vi "Calculate Directions.vi"(8 "error in (no error)":errorcluster, 10 "Heading":T1, 11 "Grassfire 2D In":refnum<class "Grassfire 2D.lvclass">) -> (0 "error out":errorcluster, 2 "Directions":T1[](array[typedef]), 3 "Grassfire 2D Out":refnum<class "Grassfire 2D.lvclass">)   [LabVIEW 2019, in "Grassfire 2D.lvclass"]
uses:
  Grassfire 2D.lvclass
  Shared/Direction--enum.ctl
  Node Address--cluster.ctl
  Grassfire 2D.lvclass/Grassfire 2D.ctl
  Shared/Node Type--enum.ctl
  <userlib>/_OpenG.lib/array/array.llb/Sort 1D Array (I32)__ogtk.vi
  <userlib>/_OpenG.lib/array/array.llb/Reorder 1D Array2 (I16)__ogtk.vi
  Shared/Shared.lvlib
panel:
  out "i":i32
  out "Total Time":u32
  out "Iteration Time":u32
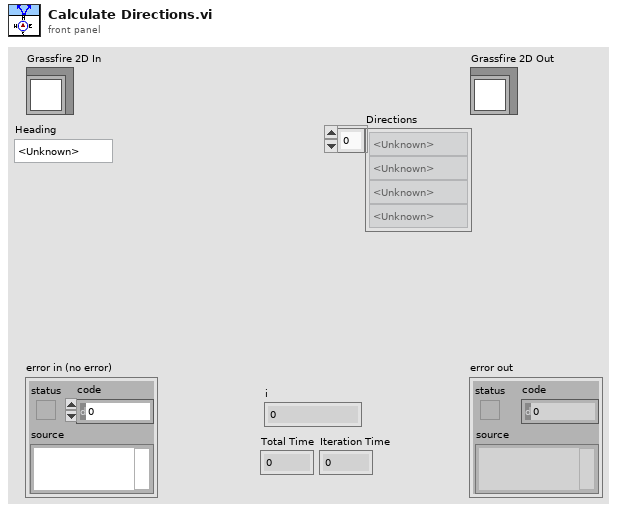
[diagram p1: front panel]
types:
  T1 = typedef "Shared.lvlib/Direction--enum.ctl" = enum16{"<Unknown>", "Right", "Down", "Left", "Up"}
  T2 = typedef "Grassfire 2D.lvclass/Node Address--cluster.ctl" = cluster{"Row":i32, "Column":i32}
  T3 = typedef "Grassfire 2D.lvclass/Node Value--cluster.ctl" = cluster{"Type":T4, "Distance":i32}
  T4 = typedef "Shared.lvlib/Node Type--enum.ctl" = enum16{"Empty", "Blocked", "Start", "End", "Path"}
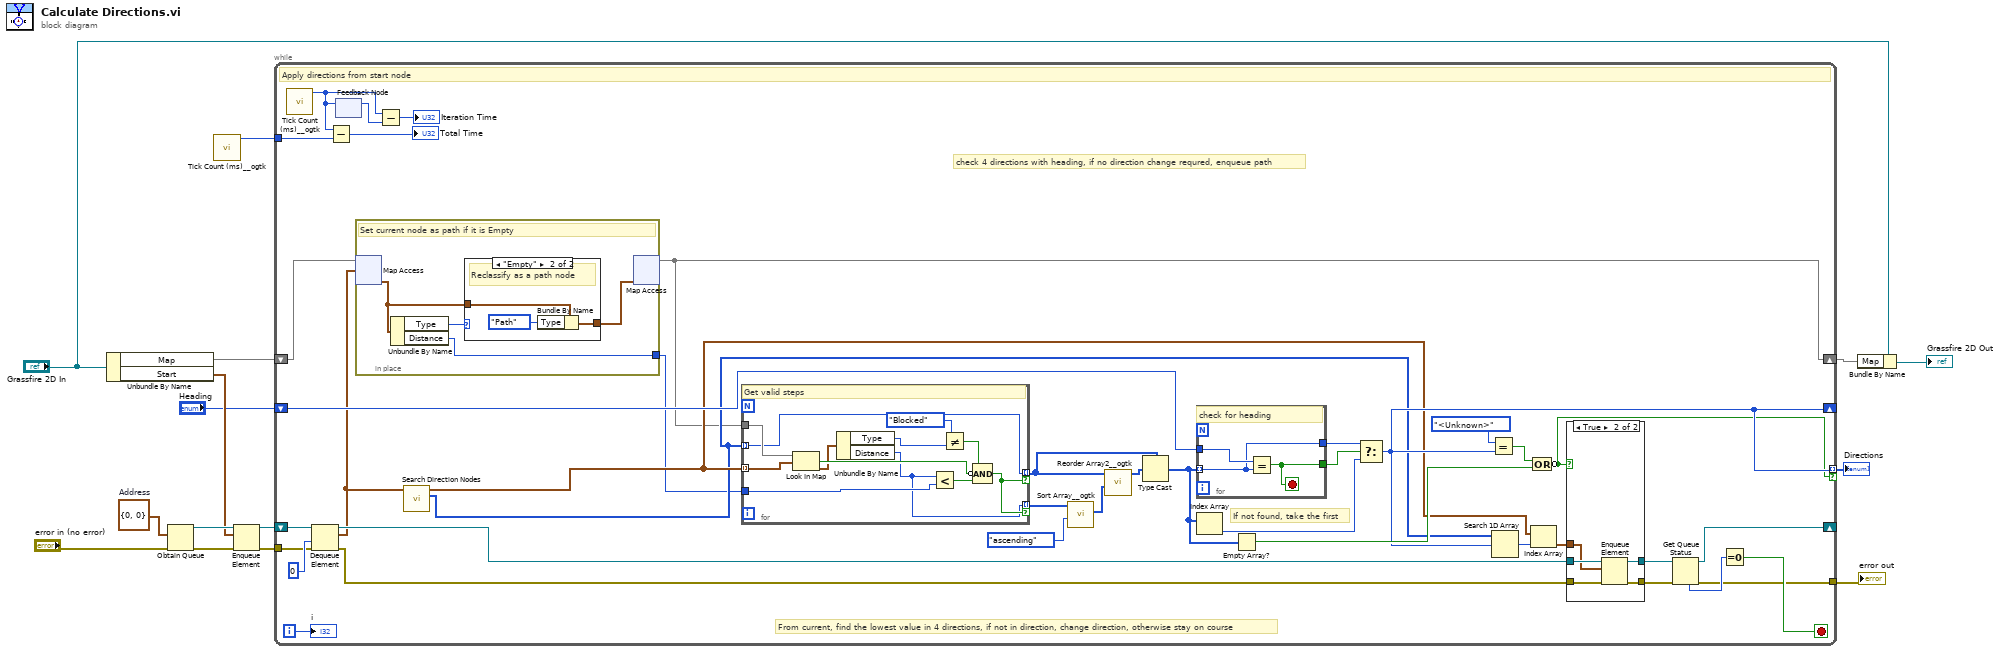
[diagram p0: block diagram]
diagram:
  w3 = T2 {"Row"=0, "Column"=0}  # Address
  n1 = Unbundle By Name("Grassfire 2D In") -> ("Map"=w12:map{T2, T3}, "Start"=w11:T2)
  n2 = Obtain Queue(element data type=w3, error in (no error)="error in (no error)") -> (queue out=w14:refnum<queue>, error out=w15:errorcluster)  [unwired: 3 in, 1 out]
  n3 = call <userlib>:"Tick Count (ms)__ogtk.vi"() -> ("millisecond timer value"=w2:u32)  [unwired: 10 in, 1 out]
  n4 = Enqueue Element(queue=w14, element=w11, error in (no error)=w15) -> (queue out=w10:refnum<queue>, error out=w9:errorcluster)  [unwired: 1 in, 1 out]
  n5 = while {
    shift-right: [w16] -> w6
    shift-left: w12 -> [w19]
    shift-right: [w51] -> _
    shift-left: w10 -> [w53]
    tunnel: w9 -> [w54]
    tunnel: [w34] -> w8
    shift-right: [w32] -> _
    shift-left: "Heading" -> [w33]
    tunnel: [w32] -> w4 mode=indexing if=w31
    tunnel: w2 -> [w21]
    i -> [w20]
    stop <- w50 stop-if-true
    # "check 4 directions with heading, if no direction change requred, enqueue path"
    # "If not found, take the first"
    # "From current, find the lowest value in 4 directions, if not in direction, change direction, otherwise stay on course"
    # "Apply directions from start node"
    n6 = call <userlib>:"Tick Count (ms)__ogtk.vi"() -> ("millisecond timer value"=w22:u32)  [unwired: 10 in, 1 out]
    n7 = Dequeue Element(queue=w53, timeout in ms (-1)=0, error in (no error)=w54) -> (queue out=w52:refnum<queue>, element=w18:T2, error out=w27:errorcluster)  [unwired: 1 out]
    n8 = Subtract(x=w22, y=w21) -> (x-y=→"Total Time":u32)
    n9 = feedback #1() -> (w24:u32)  [unwired: 1 in]
    n10 = feedback-in #1(w22) -> ()
    n11 = in-place {
      in-place-border: [w56] -> w17
      # "Set current node as path if it is Empty"
      n12 = in-place-map #2(w19, w18) -> (w58:T3)  [unwired: 1 in, 1 out]
      n13 = Unbundle By Name(w58) -> ("Type"=w57:T4, "Distance"=w56:i32)
      n14 = case shown="\"Empty\"" w57 {
        tunnel: w58 -> [w60 w63]
        tunnel: [w60 w61] -> w59
        frame Default {
          # "No Modifications"
        }
        frame "Empty" {
          # "Reclassify as a path node"
          n15 = Bundle By Name(cluster=w63, "Type"=Node_Type--enum."Path") -> (w61:T3)
        }
      }
      n16 = in-place-map #2(w59) -> (w16:map{T2, T3})  [unwired: 1 in, 2 out]
    }
    n17 = Subtract(x=w22, y=w24) -> (x-y=→"Iteration Time":u32)
    n18 = call "Search Direction Nodes.vi"("Address"=w18) -> ("Search Directions"=w28:T1[], "Search Direction Nodes"=w29:T2[])  [unwired: 9 in]
    n19 = for {
      tunnel: w16 -> [w85]
      tunnel: w29 -> [w84] mode=indexing
      tunnel: [w74] -> w48 mode=indexing if=w82
      tunnel: [w83] -> w26 mode=indexing if=w82
      tunnel: w28 -> [w83] mode=indexing
      tunnel: w17 -> [w80]
      # "Get valid steps"
      n20 = Look In Map(map=w85, key=w84) -> (key not found?=w79:bool, value=w76:T3)  [unwired: 1 in]
      n21 = Unbundle By Name(w76) -> ("Type"=w75:T4, "Distance"=w74:i32)
      n22 = Less?(x=w74, y=w80) -> (x < y?=w81:bool)
      n23 = Not Equal?(x=Node_Type--enum."Blocked" ("Selection"), y=w75) -> (x != y?=w77:bool)
      n24 = Compound Arithmetic op=AND(w77, invert w79, w81) -> (w82:bool)
    }
    n25 = call-poly <userlib>:"Sort Array__ogtk.vi"("Order"=enum16{"ascending", "descending"}."ascending", "Array in"=w48) -> ("Sorted Pointers"=w46:i32[])  [unwired: 8 in, 1 out]
    n26 = call-poly <userlib>:"Reorder Array2__ogtk.vi"("indices"=w46, "array"=w26) -> ("reordered array"=w45:i16[])  [unwired: 9 in]
    n27 = Type Cast(type=w26, x=w45) -> (*(type *) &x=w37:T1[])
    n28 = for {
      tunnel: w37 -> [w72] mode=indexing
      tunnel: w33 -> [w73]
      tunnel: [w72] -> w36
      tunnel: [w71] -> w38
      stop <- w71 stop-if-true
      # "check for heading"
      n29 = Equal?(x=w73, y=w72) -> (x = y?=w71:bool)
    }
    n30 = Index Array(array=w37) -> (element=w35:T1)  [unwired: 1 in]
    n31 = Empty Array?(array=w37) -> (empty?=w43:bool)
    n32 = Select(t=w36, s=w38, f=w35) -> (s? t:f=w32:T1)
    n33 = Equal?(x=Direction--enum."<Unknown>" ("Direction"), y=w32) -> (x = y?=w44:bool)
    n34 = Search 1D Array(1D array=w28, element=w32) -> (index of element=w42:i32)  [unwired: 1 in]
    n35 = Index Array(array=w29, index=w42) -> (element=w39:T2)
    n36 = Compound Arithmetic op=OR(w44, w43) -> (invert w31:bool)
    n37 = case shown="True" w31 {
      tunnel: w52 -> [w65 w70]
      tunnel: w27 -> [w64 w69]
      tunnel: [w65 w68] -> w41
      tunnel: [w64 w67] -> w40
      tunnel: w39 -> [_ w66]
      frame False {
      }
      frame True {
        n38 = Enqueue Element(queue=w70, element=w66, error in (no error)=w69) -> (queue out=w68:refnum<queue>, error out=w67:errorcluster)  [unwired: 1 in, 1 out]
      }
    }
    n39 = Get Queue Status(queue=w41, error in (no error)=w40) -> (queue out=w51:refnum<queue>, error out=w34:errorcluster, # elements in queue=w49:i32)  [unwired: 1 in, 5 out]
    n40 = Equal To 0?(x=w49) -> (x = 0?=w50:bool)
    "i" <- w20
  }
  "error out" <- w8
  "Directions" <- w4
  n41 = Bundle By Name(cluster="Grassfire 2D In", "Map"=w6) -> (→"Grassfire 2D Out":refnum<class "Grassfire 2D.lvclass">)
